vi "PKYK_State_Queue.vi"(8 "error in (no error)":errorcluster, 9 "PKYK_Data In":T1, 10 "State In":T5, 11 "Queue In":refnum<queue>) -> (0 "error out":errorcluster, 1 "PKYK_Data Out":T1, 3 "Queue out":refnum<queue>)   [LabVIEW 2020]
uses:
  Controls/PKYK_qData.ctl
  Controls/Poka_Status.ctl
  Controls/PKYK_Barcode_Status.ctl
  Controls/PKYK_Status.ctl
  Controls/WIP_State.ctl
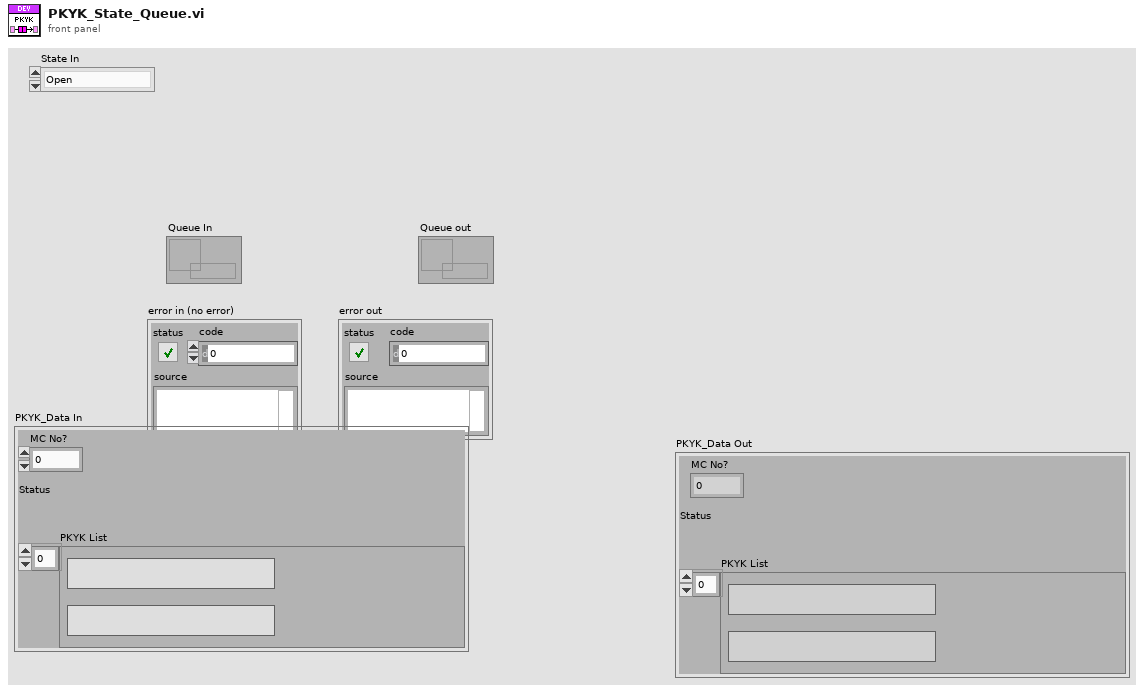
[diagram p1: front panel]
types:
  T1 = typedef "PKYK_qData.ctl" = cluster{"MC No?":i32, "Status":T2, "PKYK List":T3[]}
  T2 = typedef "Poka_Status.ctl" = u16
  T3 = typedef "PKYK_Barcode_Status.ctl" = cluster{"RFID Written Last":string, "Result":T4, "Exp. Result":T4}
  T4 = typedef "PKYK_Status.ctl" = u16
  T5 = typedef "WIP_State.ctl" = enum16{"Open", "Read", "Write", "Read WIP", "Flush", "Close"}
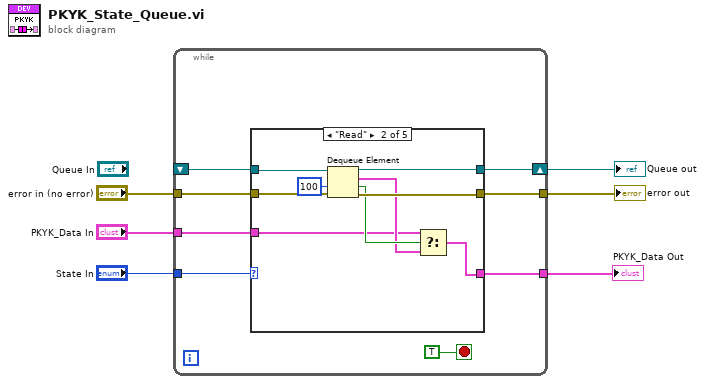
[diagram p0: block diagram]
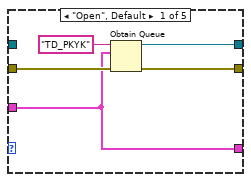
[diagram p2: hidden frame]
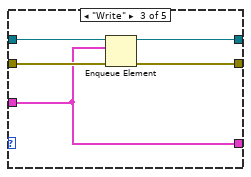
[diagram p3: hidden frame]
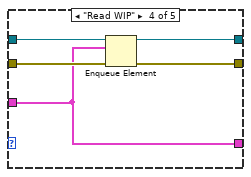
[diagram p4: hidden frame]
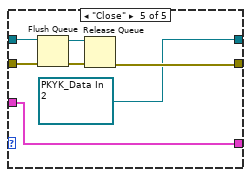
[diagram p5: hidden frame]
diagram:
  n1 = while {
    tunnel: "State In" -> [w10]
    shift-right: [w13] -> w5
    shift-left: _ -> [w9]
    tunnel: "error in (no error)" -> [w12]
    tunnel: [w14] -> w6
    tunnel: [w8] -> w1
    tunnel: "PKYK_Data In" -> [w7]
    stop <- TRUE stop-if-true
    n2 = case shown="\"Read\"" w10 {
      tunnel: [w19 w25 w30 w35 w41] -> w14
      tunnel: [w18 w24 w31 w36 refnum<queue> refnum ("Queue In")] -> w13
      tunnel: w12 -> [w16 w28 w32 w37 w45]
      tunnel: w9 -> [_ w27 w33 w38 w44]
      tunnel: [w15 w21 w29 w34 w39] -> w8
      tunnel: w7 -> [w15 w20 w29 w34 w39]
      frame "Open", Default {
        n3 = Obtain Queue(name (unnamed)="TD_PKYK", element data type=w15, error in (no error)=w16) -> (queue out=w18:refnum<queue>, error out=w19:errorcluster)  [unwired: 2 in, 1 out]
      }
      frame "Read" {
        n4 = Dequeue Element(queue=w27, timeout in ms (-1)=100, error in (no error)=w28) -> (queue out=w24:refnum<queue>, element=w22:T1, timed out?=w23:bool, error out=w25:errorcluster)
        n5 = Select(t=w20, s=w23, f=w22) -> (s? t:f=w21:T1)
      }
      frame "Write" {
        n6 = Enqueue Element(queue=w33, element=w29, error in (no error)=w32) -> (queue out=w31:refnum<queue>, error out=w30:errorcluster)  [unwired: 1 in, 1 out]
      }
      frame "Read WIP" {
        n7 = Enqueue Element(queue=w38, element=w34, error in (no error)=w37) -> (queue out=w36:refnum<queue>, error out=w35:errorcluster)  [unwired: 1 in, 1 out]
      }
      frame "Close" {
        n8 = Flush Queue(queue=w44, error in (no error)=w45) -> (queue out=w42:refnum<queue>, error out=w43:errorcluster)  [unwired: 1 out]
        n9 = Release Queue(queue=w42, error in (no error)=w43) -> (error out=w41:errorcluster)  [unwired: 1 in, 2 out]
      }
    }
  }
  "error out" <- w6
  "Queue out" <- w5
  "PKYK_Data Out" <- w1
